vi "Refresh Example Description.vi"() -> ()   [LabVIEW 2017, in "csmdoc.lvlib"]
uses:
  csmdoc.lvlib
panel:
  in  "pattern":string="VI Description(CN) - *"
  in  "LANG ID":string="CＮ"
  in  "VI":path=path "D:/CSM Framework/Communicable-State-Machine/src/user.lib/_NEVSTOP/Communicable State Machine(CSM)/Parse State Queue++.vi"
  in  "Error in":errorcluster caption="error in (no error)"
  out "error out":errorcluster
  in  "doc":path=path "D:/CSM Framework/Communicable-State-Machine/src/help/NEVSTOP/Communicable State Machine(CSM)"
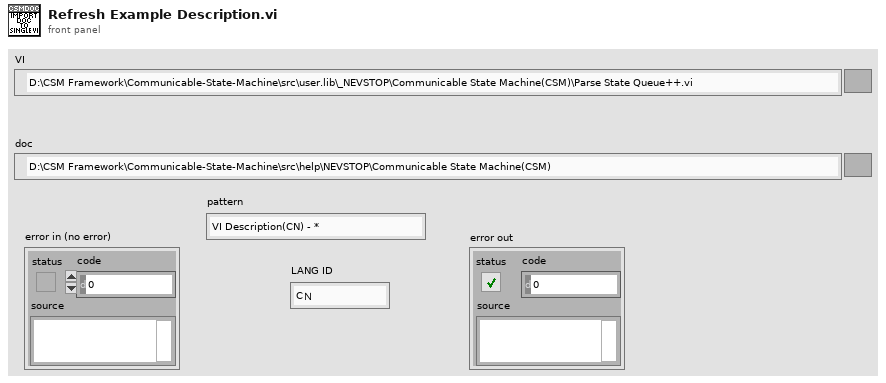
[diagram p1: front panel]
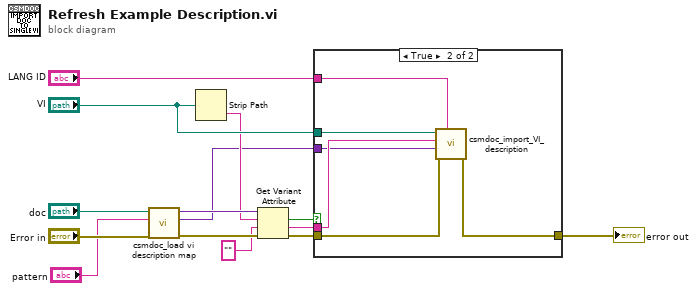
[diagram p0: block diagram]
diagram:
  n1 = call "csmdoc_load vi description map.vi"("Error In"="Error in", "Pattern"="pattern", "Path"="doc") -> ("error out"=w12:errorcluster, "NoteMap"=w3:variant, "DescMap"=w14:variant)  [unwired: 6 in]
  n2 = Strip Path(path="VI") -> (name=w8:string)  [unwired: 1 out]
  n3 = Get Variant Attribute(Variant=w14, name=w8, default value (empty Variant)="" ("String"), error in=w12) -> (found=w7:bool, value=w4:string, error out=w6:errorcluster)  [unwired: 1 out]
  n4 = case shown="True" w7 {
    tunnel: "VI" -> [_ w21]
    tunnel: w6 -> [w15 w20]
    tunnel: [w15 w19] -> w11
    tunnel: w4 -> [_ w18]
    tunnel: w3 -> [_ w17]
    tunnel: "LANG ID" -> [_ w16]
    frame False {
    }
    frame True {
      n5 = call "csmdoc_import_VI_description.vi"("LANG ID"=w16, "error in (no error)"=w20, "NOTE-Map"=w17, "String"=w18, "Path"=w21) -> ("error out"=w19:errorcluster)  [unwired: 6 in]
    }
  }
  "error out" <- w11
